vi "solar_voy_def Strip Description.vi"(11 "Name String":string) -> (2 "Description":string, 3 "Fixed Name":string)   [LabVIEW 2018]
doc: "Seperates a string into a name and a description separated by \",d=\"."
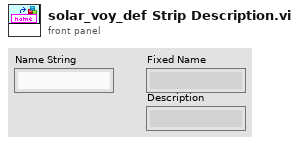
[diagram p1: front panel]
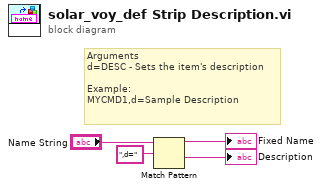
[diagram p0: block diagram]
diagram:
  # "Arguments\nd=DESC - Sets the item's description\n\nExample: \nMYCMD1,d=Sample Description"
  n1 = Match Pattern(string="Name String", regular expression=",d=" ("search string/char (-)")) -> (before substring=→"Fixed Name":string, after substring=→"Description":string)  [unwired: 1 in, 2 out]
